vi "STAT2 decode ALL Digital.vi"(0 "Received(T)":bool=TRUE, 5 "Selected Tool":T1, 7 "Controller SATT 2":T4 {"Tension Sub 2"."sys register" format="%04x"; "Tension Sub 1"."sys register" format="%04x"; "PSU"."sys register" format="%04x"; "solonoid"."valve status" format="%02x"; "solonoid"."sys register" format="%04x"; "pressure 2"."sys register" format="%04x"; "pressure 1"."sys register" format="%04x"; "Controller local"."High G monitoring" format="%02x"; "Controller local"."NA" format="%02x"; "Controller local"."GPIO values" format="%02x"; "Controller local"."Relay status" format="%02x"; "Controller local"."sys register" format="%04x"}, 9 "Analog for digital calc":T2, 11 "error in (no error)":errorcluster) -> (6 "Tool digital value":T3[](array[typedef]), 10 "Tool digital indexes":u16[](array[numeric]), 15 "error out":errorcluster)   [LabVIEW 2011]
uses:
  Stroker/Stat def/Stroker system stat2.ctl
  LEINmaster/Nodes/Controller local stat2.ctl
  LEINmaster/Nodes/pressure stat2.ctl
  LEINmaster/Nodes/solonoid stat2.ctl
  LEINmaster/Nodes/PSU stat2.ctl
  LEINmaster/Nodes/tensionsub stat2.ctl
  Measurments Handling/Status Digitalish.ctl
  Analog values for digital calculations.ctl
  List of tools.ctl
  Variable List Tool Digital.ctl
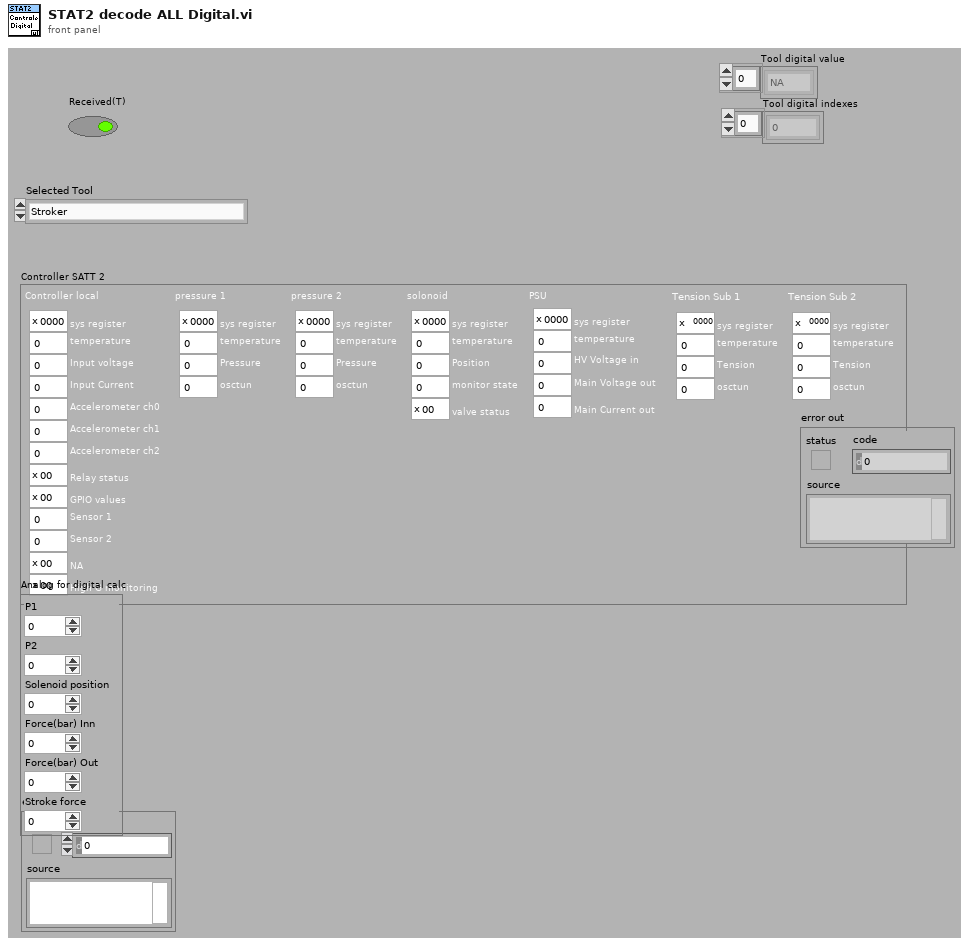
[diagram p1: front panel]
types:
  T1 = typedef "List of tools.ctl" = enum16{"Stroker", "Driller", "Tractor"}
  T2 = typedef "Analog values for digital calculations.ctl" = cluster{"P1":dbl, "P2":dbl, "Solenoid position":dbl, "Force(bar) Inn":dbl, "Force(bar) Out":dbl, "Stroke force":dbl}
  T3 = typedef "Status Digitalish.ctl" = enum16{"NA", "False", "True"}
  T4 = typedef "Stroker system stat2.ctl" = cluster{"Controller local":T5, "pressure 1":T6, "pressure 2":T6, "solonoid":T7, "PSU":T8, "Tension Sub 1":T9, "Tension Sub 2":T9}
  T5 = typedef "Controller local stat2.ctl" = cluster{"sys register":u16, "temperature":u16, "Input voltage":u16, "Input Current":u16, "Accelerometer ch0":u16, "Accelerometer ch1":u16, "Accelerometer ch2":u16, "Relay status":u8, "GPIO values":u8, "Sensor 1":i32, "Sensor 2":i32, "NA":u8, "High G monitoring":u8}
  T6 = typedef "pressure stat2.ctl" = cluster{"sys register":u16, "temperature":u16, "Pressure":u16, "osctun":u8}
  T7 = typedef "solonoid stat2.ctl" = cluster{"sys register":u16, "temperature":u16, "Position":i16, "monitor state":u8, "valve status":u8}
  T8 = typedef "PSU stat2.ctl" = cluster{"sys register":u16, "temperature":u16, "HV Voltage in":u16, "Main Voltage out":u16, "Main Current out":u16}
  T9 = typedef "tensionsub stat2.ctl" = cluster{"sys register":u16, "temperature":u16, "Tension":i16, "osctun":u8}
  T10 = typedef "Variable List Tool Digital.ctl" = enum16{"Tool Error Controller", "Tool Stopped Controller", "Tool Relay 1", "Tool Relay 2", "Tool Both Relays", "Tool node Pressure 1", "Tool Error Pressure 1", "Tool Stopped Pressure 1", "Tool node Pressure 2", "Tool Error Pressure 2", "Tool Stopped Pressure 2", "Tool node Solenoid", "Tool Error Solenoid", "Tool Stopped Solenoid", "Tool Solenoid 1", "Tool Solenoid 2", "Tool Solenoid 3", "Tool node PSU", "Tool Error PSU", "Tool Stopped PSU", "Upper Tension Sub", "Tool Error Upper Tension Sub", "Tool Stopped Upper Tension Sub", "Lower Tension Sub", "Tool Error Lower Tension Sub", "Tool Stopped Lower Tension Sub", "Stroke Target seeking", "Stroke Moving Out", "Stroke Moving Inn", "Stroke valves set for Out", "Stroke valves set for In", "Stroke In (force)", "Stroke Out (force)", "Stroke Force decreasing(in)", "Stroke Force decreasing(out)", "Stroke Force change not correct", "Stroke SLIPS established P1", "Stroke SLIPS established P2", "Stroke SLIPS established", "Stroke Pressure Monitor Ongoing", "Stroke Pressure Monitor Ending ", "Tool Stroke enable Valve", "Tool Stroke direction Valve", "Tool Anchor Valve", "Stroker Var19 - Reserved", "Stroker Var20 - Reserved", "Stroker Var21 - Reserved", "Stroker Var22 - Reserved", "Stroker Var23 - Reserved", "Stroker Var24 - Reserved", "Tractor Var1 - Reserved", "Tractor Var2 - Reserved", "Tractor Var3 - Reserved", "Tractor Var4 - Reserved", "Tractor Var5 - Reserved", "Tractor Var6 - Reserved", "Tractor Var7 - Reserved", "Tractor Var8 - Reserved", "Oil filling mode", "Mill Bit Direction", "Position control", "Anchor", "Driller Var5 - Reserved", "Driller Var6 - Reserved", "Driller Var7 - Reserved", "Driller Var8 - Reserved"}
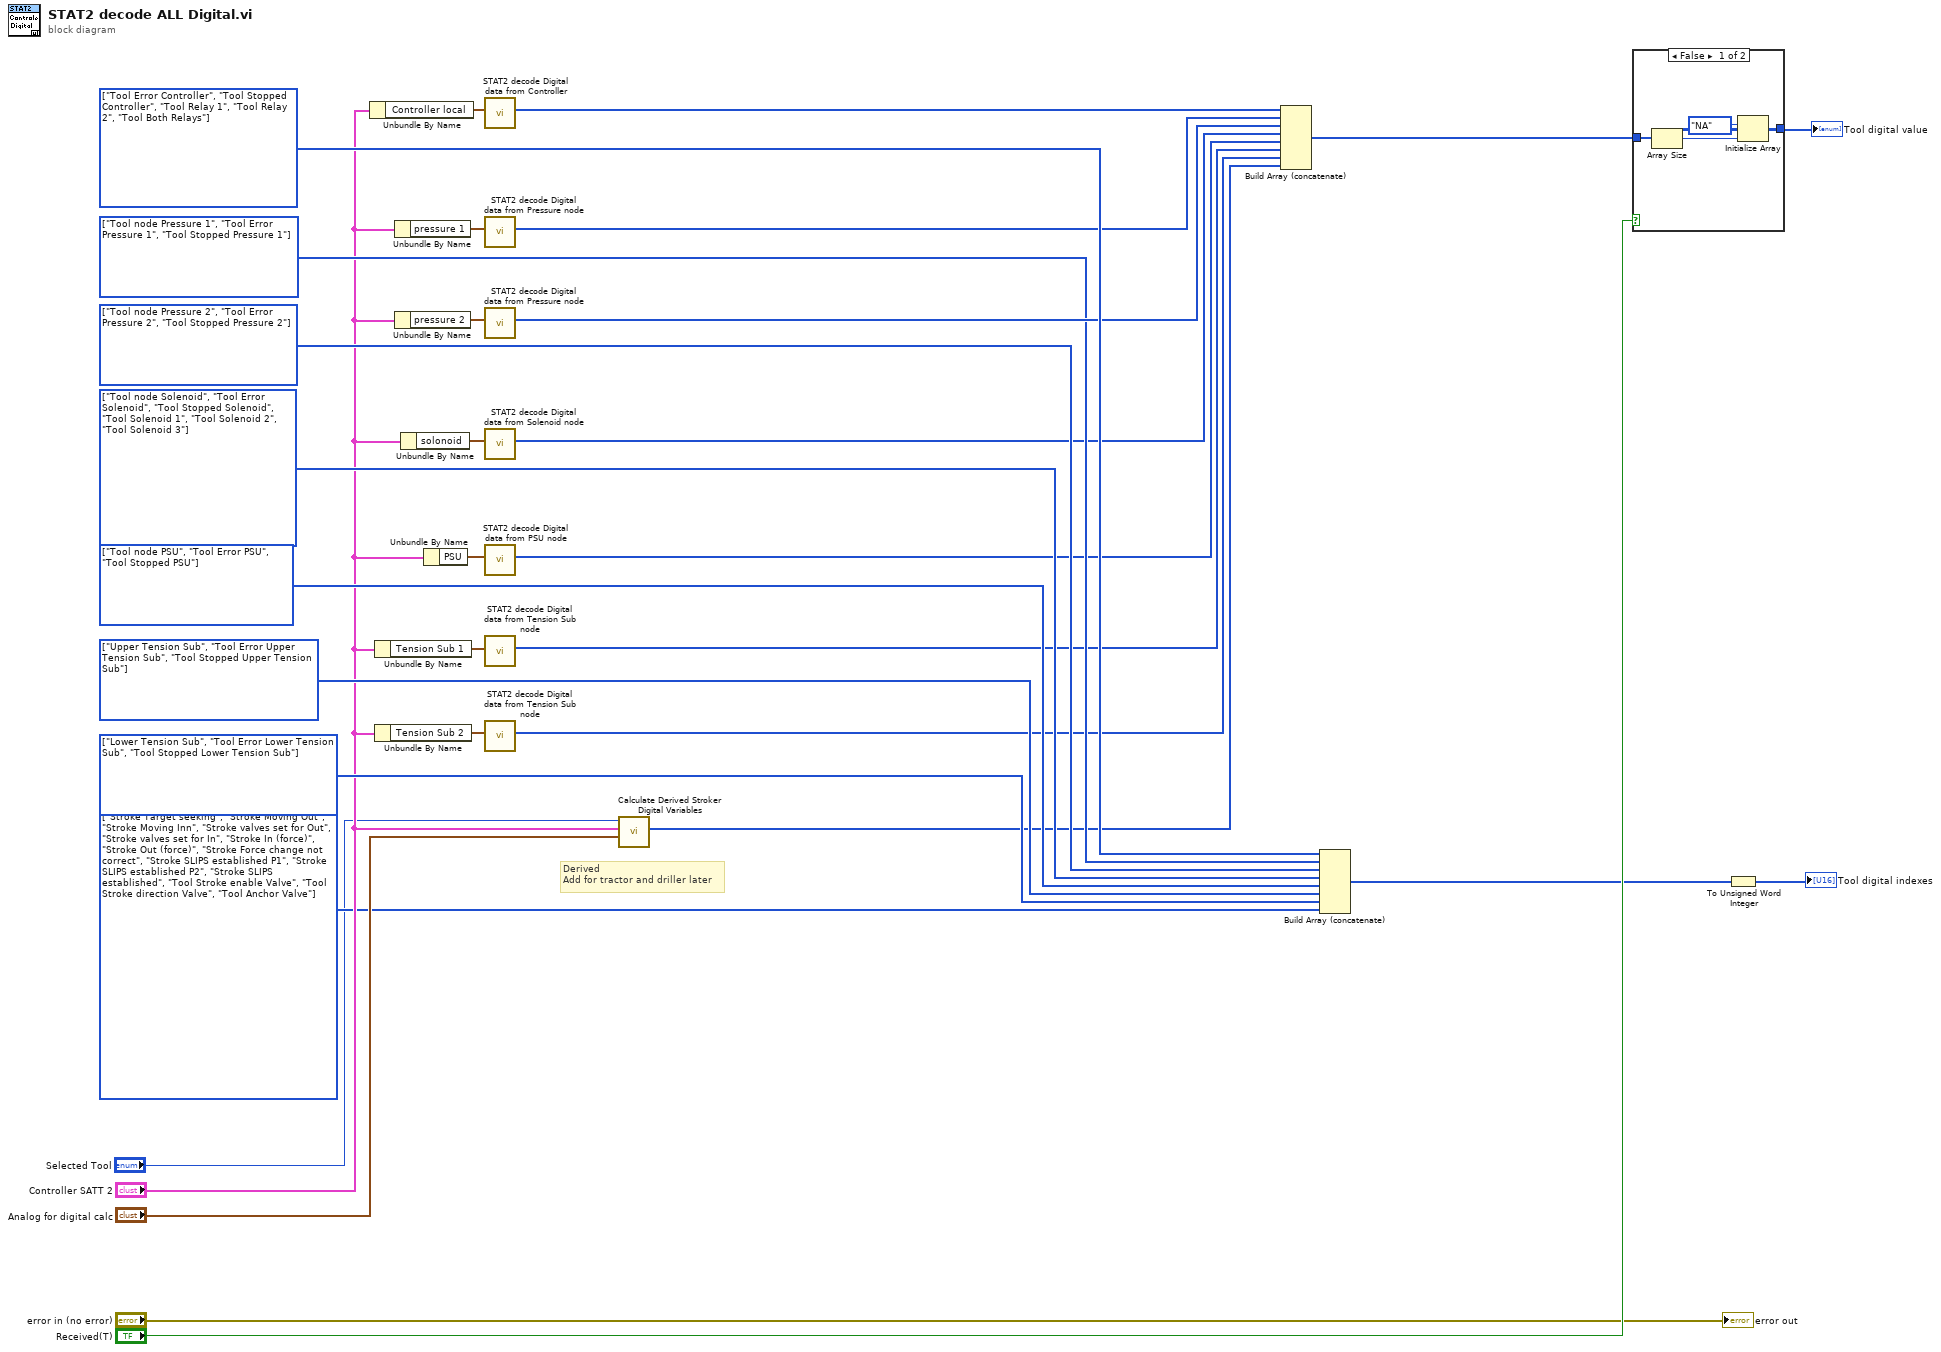
[diagram p0: block diagram]
diagram:
  w2 = T10[] [enum."Stroke Target seeking", enum."Stroke Moving Out", enum."Stroke Moving Inn", enum."Stroke valves set for Out", enum."Stroke valves set for In", enum."Stroke In (force)", enum."Stroke Out (force)", enum."Stroke Force change not correct", enum."Stroke SLIPS established P1", enum."Stroke SLIPS established P2", enum."Stroke SLIPS established", enum."Tool Stroke enable Valve", enum."Tool Stroke direction Valve", enum."Tool Anchor Valve"] items=["Tool Error Controller", "Tool Stopped Controller", "Tool Relay 1", "Tool Relay 2", "Tool Both Relays", "Tool node Pressure 1", "Tool Error Pressure 1", "Tool Stopped Pressure 1", "Tool node Pressure 2", "Tool Error Pressure 2", "Tool Stopped Pressure 2", "Tool node Solenoid", "Tool Error Solenoid", "Tool Stopped Solenoid", "Tool Solenoid 1", "Tool Solenoid 2", "Tool Solenoid 3", "Tool node PSU", "Tool Error PSU", "Tool Stopped PSU", "Upper Tension Sub", "Tool Error Upper Tension Sub", "Tool Stopped Upper Tension Sub", "Lower Tension Sub", "Tool Error Lower Tension Sub", "Tool Stopped Lower Tension Sub", "Stroke Target seeking", "Stroke Moving Out", "Stroke Moving Inn", "Stroke valves set for Out", "Stroke valves set for In", "Stroke In (force)", "Stroke Out (force)", "Stroke Force decreasing(in)", "Stroke Force decreasing(out)", "Stroke Force change not correct", "Stroke SLIPS established P1", "Stroke SLIPS established P2", "Stroke SLIPS established", "Stroke Pressure Monitor Ongoing", "Stroke Pressure Monitor Ending ", "Tool Stroke enable Valve", "Tool Stroke direction Valve", "Tool Anchor Valve", "Stroker Var19 - Reserved", "Stroker Var20 - Reserved", "Stroker Var21 - Reserved", "Stroker Var22 - Reserved", "Stroker Var23 - Reserved", "Stroker Var24 - Reserved", "Tractor Var1 - Reserved", "Tractor Var2 - Reserved", "Tractor Var3 - Reserved", "Tractor Var4 - Reserved", "Tractor Var5 - Reserved", "Tractor Var6 - Reserved", "Tractor Var7 - Reserved", "Tractor Var8 - Reserved", "Oil filling mode", "Mill Bit Direction", "Position control", "Anchor", "Driller Var5 - Reserved", "Driller Var6 - Reserved", "Driller Var7 - Reserved", "Driller Var8 - Reserved"]
  w11 = T10[] [enum."Lower Tension Sub", enum."Tool Error Lower Tension Sub", enum."Tool Stopped Lower Tension Sub"] items=["Tool Error Controller", "Tool Stopped Controller", "Tool Relay 1", "Tool Relay 2", "Tool Both Relays", "Tool node Pressure 1", "Tool Error Pressure 1", "Tool Stopped Pressure 1", "Tool node Pressure 2", "Tool Error Pressure 2", "Tool Stopped Pressure 2", "Tool node Solenoid", "Tool Error Solenoid", "Tool Stopped Solenoid", "Tool Solenoid 1", "Tool Solenoid 2", "Tool Solenoid 3", "Tool node PSU", "Tool Error PSU", "Tool Stopped PSU", "Upper Tension Sub", "Tool Error Upper Tension Sub", "Tool Stopped Upper Tension Sub", "Lower Tension Sub", "Tool Error Lower Tension Sub", "Tool Stopped Lower Tension Sub", "Stroke Target seeking", "Stroke Moving Out", "Stroke Moving Inn", "Stroke valves set for Out", "Stroke valves set for In", "Stroke In (force)", "Stroke Out (force)", "Stroke Force decreasing(in)", "Stroke Force decreasing(out)", "Stroke Force change not correct", "Stroke SLIPS established P1", "Stroke SLIPS established P2", "Stroke SLIPS established", "Stroke Pressure Monitor Ongoing", "Stroke Pressure Monitor Ending ", "Tool Stroke enable Valve", "Tool Stroke direction Valve", "Tool Anchor Valve", "Stroker Var19 - Reserved", "Stroker Var20 - Reserved", "Stroker Var21 - Reserved", "Stroker Var22 - Reserved", "Stroker Var23 - Reserved", "Stroker Var24 - Reserved", "Tractor Var1 - Reserved", "Tractor Var2 - Reserved", "Tractor Var3 - Reserved", "Tractor Var4 - Reserved", "Tractor Var5 - Reserved", "Tractor Var6 - Reserved", "Tractor Var7 - Reserved", "Tractor Var8 - Reserved", "Oil filling mode", "Mill Bit Direction", "Position control", "Anchor", "Driller Var5 - Reserved", "Driller Var6 - Reserved", "Driller Var7 - Reserved", "Driller Var8 - Reserved"]
  w12 = T10[] [enum."Upper Tension Sub", enum."Tool Error Upper Tension Sub", enum."Tool Stopped Upper Tension Sub"] items=["Tool Error Controller", "Tool Stopped Controller", "Tool Relay 1", "Tool Relay 2", "Tool Both Relays", "Tool node Pressure 1", "Tool Error Pressure 1", "Tool Stopped Pressure 1", "Tool node Pressure 2", "Tool Error Pressure 2", "Tool Stopped Pressure 2", "Tool node Solenoid", "Tool Error Solenoid", "Tool Stopped Solenoid", "Tool Solenoid 1", "Tool Solenoid 2", "Tool Solenoid 3", "Tool node PSU", "Tool Error PSU", "Tool Stopped PSU", "Upper Tension Sub", "Tool Error Upper Tension Sub", "Tool Stopped Upper Tension Sub", "Lower Tension Sub", "Tool Error Lower Tension Sub", "Tool Stopped Lower Tension Sub", "Stroke Target seeking", "Stroke Moving Out", "Stroke Moving Inn", "Stroke valves set for Out", "Stroke valves set for In", "Stroke In (force)", "Stroke Out (force)", "Stroke Force decreasing(in)", "Stroke Force decreasing(out)", "Stroke Force change not correct", "Stroke SLIPS established P1", "Stroke SLIPS established P2", "Stroke SLIPS established", "Stroke Pressure Monitor Ongoing", "Stroke Pressure Monitor Ending ", "Tool Stroke enable Valve", "Tool Stroke direction Valve", "Tool Anchor Valve", "Stroker Var19 - Reserved", "Stroker Var20 - Reserved", "Stroker Var21 - Reserved", "Stroker Var22 - Reserved", "Stroker Var23 - Reserved", "Stroker Var24 - Reserved", "Tractor Var1 - Reserved", "Tractor Var2 - Reserved", "Tractor Var3 - Reserved", "Tractor Var4 - Reserved", "Tractor Var5 - Reserved", "Tractor Var6 - Reserved", "Tractor Var7 - Reserved", "Tractor Var8 - Reserved", "Oil filling mode", "Mill Bit Direction", "Position control", "Anchor", "Driller Var5 - Reserved", "Driller Var6 - Reserved", "Driller Var7 - Reserved", "Driller Var8 - Reserved"]
  w14 = T10[] [enum."Tool node PSU", enum."Tool Error PSU", enum."Tool Stopped PSU"] items=["Tool Error Controller", "Tool Stopped Controller", "Tool Relay 1", "Tool Relay 2", "Tool Both Relays", "Tool node Pressure 1", "Tool Error Pressure 1", "Tool Stopped Pressure 1", "Tool node Pressure 2", "Tool Error Pressure 2", "Tool Stopped Pressure 2", "Tool node Solenoid", "Tool Error Solenoid", "Tool Stopped Solenoid", "Tool Solenoid 1", "Tool Solenoid 2", "Tool Solenoid 3", "Tool node PSU", "Tool Error PSU", "Tool Stopped PSU", "Upper Tension Sub", "Tool Error Upper Tension Sub", "Tool Stopped Upper Tension Sub", "Lower Tension Sub", "Tool Error Lower Tension Sub", "Tool Stopped Lower Tension Sub", "Stroke Target seeking", "Stroke Moving Out", "Stroke Moving Inn", "Stroke valves set for Out", "Stroke valves set for In", "Stroke In (force)", "Stroke Out (force)", "Stroke Force decreasing(in)", "Stroke Force decreasing(out)", "Stroke Force change not correct", "Stroke SLIPS established P1", "Stroke SLIPS established P2", "Stroke SLIPS established", "Stroke Pressure Monitor Ongoing", "Stroke Pressure Monitor Ending ", "Tool Stroke enable Valve", "Tool Stroke direction Valve", "Tool Anchor Valve", "Stroker Var19 - Reserved", "Stroker Var20 - Reserved", "Stroker Var21 - Reserved", "Stroker Var22 - Reserved", "Stroker Var23 - Reserved", "Stroker Var24 - Reserved", "Tractor Var1 - Reserved", "Tractor Var2 - Reserved", "Tractor Var3 - Reserved", "Tractor Var4 - Reserved", "Tractor Var5 - Reserved", "Tractor Var6 - Reserved", "Tractor Var7 - Reserved", "Tractor Var8 - Reserved", "Oil filling mode", "Mill Bit Direction", "Position control", "Anchor", "Driller Var5 - Reserved", "Driller Var6 - Reserved", "Driller Var7 - Reserved", "Driller Var8 - Reserved"]
  w16 = T10[] [enum."Tool node Solenoid", enum."Tool Error Solenoid", enum."Tool Stopped Solenoid", enum."Tool Solenoid 1", enum."Tool Solenoid 2", enum."Tool Solenoid 3"] items=["Tool Error Controller", "Tool Stopped Controller", "Tool Relay 1", "Tool Relay 2", "Tool Both Relays", "Tool node Pressure 1", "Tool Error Pressure 1", "Tool Stopped Pressure 1", "Tool node Pressure 2", "Tool Error Pressure 2", "Tool Stopped Pressure 2", "Tool node Solenoid", "Tool Error Solenoid", "Tool Stopped Solenoid", "Tool Solenoid 1", "Tool Solenoid 2", "Tool Solenoid 3", "Tool node PSU", "Tool Error PSU", "Tool Stopped PSU", "Upper Tension Sub", "Tool Error Upper Tension Sub", "Tool Stopped Upper Tension Sub", "Lower Tension Sub", "Tool Error Lower Tension Sub", "Tool Stopped Lower Tension Sub", "Stroke Target seeking", "Stroke Moving Out", "Stroke Moving Inn", "Stroke valves set for Out", "Stroke valves set for In", "Stroke In (force)", "Stroke Out (force)", "Stroke Force decreasing(in)", "Stroke Force decreasing(out)", "Stroke Force change not correct", "Stroke SLIPS established P1", "Stroke SLIPS established P2", "Stroke SLIPS established", "Stroke Pressure Monitor Ongoing", "Stroke Pressure Monitor Ending ", "Tool Stroke enable Valve", "Tool Stroke direction Valve", "Tool Anchor Valve", "Stroker Var19 - Reserved", "Stroker Var20 - Reserved", "Stroker Var21 - Reserved", "Stroker Var22 - Reserved", "Stroker Var23 - Reserved", "Stroker Var24 - Reserved", "Tractor Var1 - Reserved", "Tractor Var2 - Reserved", "Tractor Var3 - Reserved", "Tractor Var4 - Reserved", "Tractor Var5 - Reserved", "Tractor Var6 - Reserved", "Tractor Var7 - Reserved", "Tractor Var8 - Reserved", "Oil filling mode", "Mill Bit Direction", "Position control", "Anchor", "Driller Var5 - Reserved", "Driller Var6 - Reserved", "Driller Var7 - Reserved", "Driller Var8 - Reserved"]
  w17 = T10[] [enum."Tool node Pressure 2", enum."Tool Error Pressure 2", enum."Tool Stopped Pressure 2"] items=["Tool Error Controller", "Tool Stopped Controller", "Tool Relay 1", "Tool Relay 2", "Tool Both Relays", "Tool node Pressure 1", "Tool Error Pressure 1", "Tool Stopped Pressure 1", "Tool node Pressure 2", "Tool Error Pressure 2", "Tool Stopped Pressure 2", "Tool node Solenoid", "Tool Error Solenoid", "Tool Stopped Solenoid", "Tool Solenoid 1", "Tool Solenoid 2", "Tool Solenoid 3", "Tool node PSU", "Tool Error PSU", "Tool Stopped PSU", "Upper Tension Sub", "Tool Error Upper Tension Sub", "Tool Stopped Upper Tension Sub", "Lower Tension Sub", "Tool Error Lower Tension Sub", "Tool Stopped Lower Tension Sub", "Stroke Target seeking", "Stroke Moving Out", "Stroke Moving Inn", "Stroke valves set for Out", "Stroke valves set for In", "Stroke In (force)", "Stroke Out (force)", "Stroke Force decreasing(in)", "Stroke Force decreasing(out)", "Stroke Force change not correct", "Stroke SLIPS established P1", "Stroke SLIPS established P2", "Stroke SLIPS established", "Stroke Pressure Monitor Ongoing", "Stroke Pressure Monitor Ending ", "Tool Stroke enable Valve", "Tool Stroke direction Valve", "Tool Anchor Valve", "Stroker Var19 - Reserved", "Stroker Var20 - Reserved", "Stroker Var21 - Reserved", "Stroker Var22 - Reserved", "Stroker Var23 - Reserved", "Stroker Var24 - Reserved", "Tractor Var1 - Reserved", "Tractor Var2 - Reserved", "Tractor Var3 - Reserved", "Tractor Var4 - Reserved", "Tractor Var5 - Reserved", "Tractor Var6 - Reserved", "Tractor Var7 - Reserved", "Tractor Var8 - Reserved", "Oil filling mode", "Mill Bit Direction", "Position control", "Anchor", "Driller Var5 - Reserved", "Driller Var6 - Reserved", "Driller Var7 - Reserved", "Driller Var8 - Reserved"]
  w18 = T10[] [enum."Tool node Pressure 1", enum."Tool Error Pressure 1", enum."Tool Stopped Pressure 1"] items=["Tool Error Controller", "Tool Stopped Controller", "Tool Relay 1", "Tool Relay 2", "Tool Both Relays", "Tool node Pressure 1", "Tool Error Pressure 1", "Tool Stopped Pressure 1", "Tool node Pressure 2", "Tool Error Pressure 2", "Tool Stopped Pressure 2", "Tool node Solenoid", "Tool Error Solenoid", "Tool Stopped Solenoid", "Tool Solenoid 1", "Tool Solenoid 2", "Tool Solenoid 3", "Tool node PSU", "Tool Error PSU", "Tool Stopped PSU", "Upper Tension Sub", "Tool Error Upper Tension Sub", "Tool Stopped Upper Tension Sub", "Lower Tension Sub", "Tool Error Lower Tension Sub", "Tool Stopped Lower Tension Sub", "Stroke Target seeking", "Stroke Moving Out", "Stroke Moving Inn", "Stroke valves set for Out", "Stroke valves set for In", "Stroke In (force)", "Stroke Out (force)", "Stroke Force decreasing(in)", "Stroke Force decreasing(out)", "Stroke Force change not correct", "Stroke SLIPS established P1", "Stroke SLIPS established P2", "Stroke SLIPS established", "Stroke Pressure Monitor Ongoing", "Stroke Pressure Monitor Ending ", "Tool Stroke enable Valve", "Tool Stroke direction Valve", "Tool Anchor Valve", "Stroker Var19 - Reserved", "Stroker Var20 - Reserved", "Stroker Var21 - Reserved", "Stroker Var22 - Reserved", "Stroker Var23 - Reserved", "Stroker Var24 - Reserved", "Tractor Var1 - Reserved", "Tractor Var2 - Reserved", "Tractor Var3 - Reserved", "Tractor Var4 - Reserved", "Tractor Var5 - Reserved", "Tractor Var6 - Reserved", "Tractor Var7 - Reserved", "Tractor Var8 - Reserved", "Oil filling mode", "Mill Bit Direction", "Position control", "Anchor", "Driller Var5 - Reserved", "Driller Var6 - Reserved", "Driller Var7 - Reserved", "Driller Var8 - Reserved"]
  w22 = T10[] [enum."Tool Error Controller", enum."Tool Stopped Controller", enum."Tool Relay 1", enum."Tool Relay 2", enum."Tool Both Relays"] items=["Tool Error Controller", "Tool Stopped Controller", "Tool Relay 1", "Tool Relay 2", "Tool Both Relays", "Tool node Pressure 1", "Tool Error Pressure 1", "Tool Stopped Pressure 1", "Tool node Pressure 2", "Tool Error Pressure 2", "Tool Stopped Pressure 2", "Tool node Solenoid", "Tool Error Solenoid", "Tool Stopped Solenoid", "Tool Solenoid 1", "Tool Solenoid 2", "Tool Solenoid 3", "Tool node PSU", "Tool Error PSU", "Tool Stopped PSU", "Upper Tension Sub", "Tool Error Upper Tension Sub", "Tool Stopped Upper Tension Sub", "Lower Tension Sub", "Tool Error Lower Tension Sub", "Tool Stopped Lower Tension Sub", "Stroke Target seeking", "Stroke Moving Out", "Stroke Moving Inn", "Stroke valves set for Out", "Stroke valves set for In", "Stroke In (force)", "Stroke Out (force)", "Stroke Force decreasing(in)", "Stroke Force decreasing(out)", "Stroke Force change not correct", "Stroke SLIPS established P1", "Stroke SLIPS established P2", "Stroke SLIPS established", "Stroke Pressure Monitor Ongoing", "Stroke Pressure Monitor Ending ", "Tool Stroke enable Valve", "Tool Stroke direction Valve", "Tool Anchor Valve", "Stroker Var19 - Reserved", "Stroker Var20 - Reserved", "Stroker Var21 - Reserved", "Stroker Var22 - Reserved", "Stroker Var23 - Reserved", "Stroker Var24 - Reserved", "Tractor Var1 - Reserved", "Tractor Var2 - Reserved", "Tractor Var3 - Reserved", "Tractor Var4 - Reserved", "Tractor Var5 - Reserved", "Tractor Var6 - Reserved", "Tractor Var7 - Reserved", "Tractor Var8 - Reserved", "Oil filling mode", "Mill Bit Direction", "Position control", "Anchor", "Driller Var5 - Reserved", "Driller Var6 - Reserved", "Driller Var7 - Reserved", "Driller Var8 - Reserved"]
  # "Derived\nAdd for tractor and driller later"
  n1 = Unbundle By Name("Controller SATT 2") -> ("Controller local"=w29:T5)
  n2 = Unbundle By Name("Controller SATT 2") -> ("Tension Sub 1"=w24:T9)
  n3 = Unbundle By Name("Controller SATT 2") -> ("Tension Sub 2"=w23:T9)
  n4 = Unbundle By Name("Controller SATT 2") -> ("pressure 1"=w28:T6)
  n5 = Unbundle By Name("Controller SATT 2") -> ("pressure 2"=w27:T6)
  n6 = Unbundle By Name("Controller SATT 2") -> ("solonoid"=w26:T7)
  n7 = Unbundle By Name("Controller SATT 2") -> ("PSU"=w25:T8)
  n8 = call "STAT2 decode Digital data from Controller.vi"("Controller Data"=w29) -> ("Digital Data Out"=w21:T3[])  [unwired: 10 in]
  n9 = call "STAT2 decode Digital data from Pressure node.vi"("Pressure Node Data"=w28) -> ("Digital Data Out"=w20:T3[])  [unwired: 10 in]
  n10 = call "STAT2 decode Digital data from Pressure node.vi"("Pressure Node Data"=w27) -> ("Digital Data Out"=w19:T3[])  [unwired: 10 in]
  n11 = call "STAT2 decode Digital data from Solenoid node.vi"("Solenoid Node Data"=w26) -> ("Digital Data Out"=w15:T3[])  [unwired: 10 in]
  n12 = call "STAT2 decode Digital data from PSU node.vi"("PSU Node Data"=w25) -> ("Digital Data Out"=w13:T3[])  [unwired: 10 in]
  n13 = call "STAT2 decode Digital data from Tension Sub node.vi"("Tension Sub Node Data"=w24) -> ("Digital Data Out"=w10:T3[])  [unwired: 10 in]
  n14 = call "STAT2 decode Digital data from Tension Sub node.vi"("Tension Sub Node Data"=w23) -> ("Digital Data Out"=w9:T3[])  [unwired: 10 in]
  n15 = call "Calculate Derived Stroker Digital Variables.vi"("Analog for digital calc"="Analog for digital calc", "Controller STAT2"="Controller SATT 2", "Selected Tool"="Selected Tool") -> ("Digital Variables Out"=w4:T3[])  [unwired: 7 in, 1 out]
  n16 = Build Array (concatenate)(w21, w20, w19, w15, w13, w10, w9, w4) -> (w7:T3[])
  n17 = Build Array (concatenate)(w22, w18, w17, w16, w14, w12, w11, w2) -> (w3:T10[])
  n18 = case shown="False" "Received(T)" {
    tunnel: [w34 w37] -> w32
    tunnel: w7 -> [w36 w37]
    frame False {
      n19 = Array Size(array=w36) -> (size(s)=w35:i32)
      n20 = Initialize Array(Status_Digitalish."NA" ("Status"), w35) -> (w34:T3[])
    }
    frame True {
    }
  }
  "Tool digital value" <- w32
  n21 = To Unsigned Word Integer(number=w3) -> (unsigned 16bit integer=→"Tool digital indexes":u16[])
  "error out" <- "error in (no error)"
